vi "unmarshalling.vi"(7 "Type":variant, 8 "error in (no error)":errorcluster, 10 "B64 Encoded String":string, 11 "Serializer.Base64 in":refnum<class "Serializer.Base64.lvclass">) -> (0 "error out":errorcluster, 2 "Variant":variant, 3 "Serializer.Base64 out":refnum<class "Serializer.Base64.lvclass">)   [LabVIEW 2019, in "OpenSerializer.base64.lvlib" / "Serializer.Base64.lvclass"]
uses:
  Serializer.Base64.lvclass
  Base64_ByteLUT.vi
  <vilib>/LabVIEW Open Source Project/OpenSerializer/Serializer.FlattenedString/Serializer.FlattenedString.lvclass
  OpenSerializer.base64.lvlib
  <vilib>/LabVIEW Open Source Project/Data Manipulation/TypeDescriptor/OpenDescriptor.lvlib
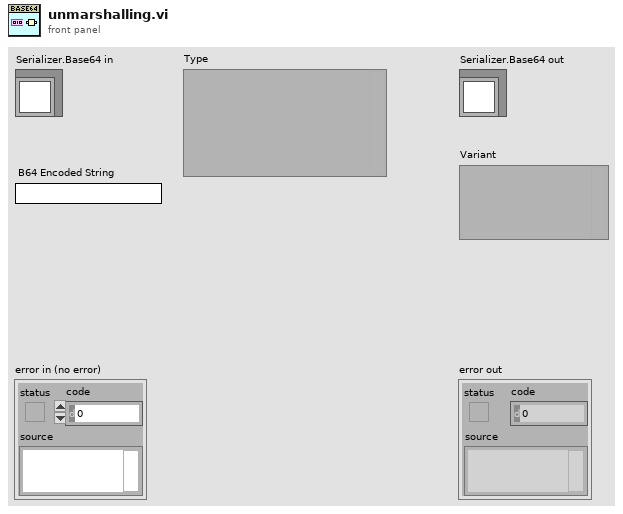
[diagram p1: front panel]
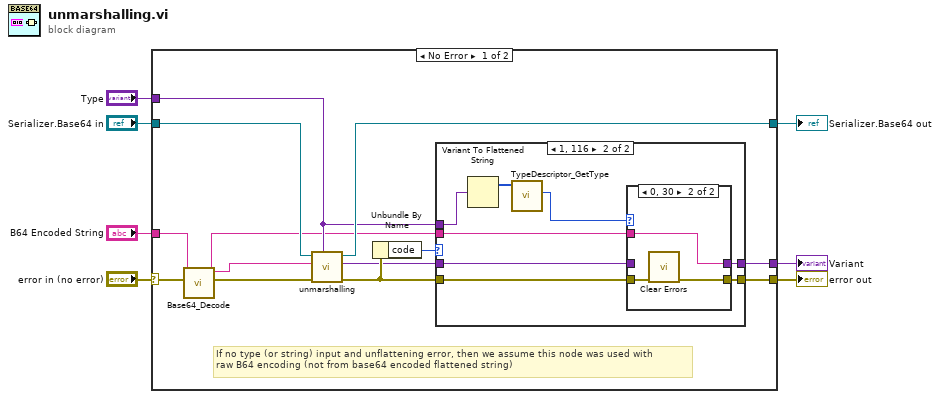
[diagram p0: block diagram]
diagram:
  n1 = case shown="No Error" "error in (no error)" {
    selector: "error in (no error)" -> [w10 w35]
    tunnel: "Serializer.Base64 in" -> [w19 w36]
    tunnel: "B64 Encoded String" -> [w9 _]
    tunnel: [w17 w36] -> w5
    tunnel: [w14 w35] -> w4
    tunnel: [w13 _] -> w3
    tunnel: "Type" -> [w11 _]
    frame No Error {
      # "If no type (or string) input and unflattening error, then we assume this node was used with\nraw B64 encoding (not from base64 encoded flattened string)"
      n2 = call "Base64_Decode.vi"("error in (no error)"=w10, "Base64 String"=w9) -> ("error out"=w18:errorcluster, "Decoded String"=w8:string)  [unwired: 8 in]
      n3 = call-parent "unmarshalling.vi"("Type"=w11, "error in (no error)"=w18, "String"=w8, "Serializer in"=w19) -> ("error out"=w15:errorcluster, "Variant"=w12:variant, "Serializer out"=w17:refnum<class "Serializer.Base64.lvclass">)  [unwired: 5 in]
      n4 = Unbundle By Name(w15) -> ("code"=w16:i32)
      n5 = case shown="1, 116" w16 {
        tunnel: w15 -> [w20 w29]
        tunnel: [w20 w28] -> w14
        tunnel: [w21 w27] -> w13
        tunnel: w12 -> [w21 w26]
        tunnel: w11 -> [_ w24]
        tunnel: w8 -> [_ w25]
        frame Default {
        }
        frame 1, 116 {
          n6 = Variant To Flattened String(Variant=w24) -> (1:w23:i16[])  [unwired: 1 out]
          n7 = call <vilib>:"TypeDescriptor_GetType.vi"("type descriptor"=w23) -> ("Type"=w22:u8)  [unwired: 9 in, 1 out]
          n8 = case shown="0, 30" w22 {
            tunnel: w29 -> [w31 w34]
            tunnel: [w31 w32] -> w28
            tunnel: [w30 w33] -> w27
            tunnel: w26 -> [w30 _]
            tunnel: w25 -> [_ w33]
            frame Default {
            }
            frame 0, 48 {
              n9 = call <vilib>:"Clear Errors.vi"("error in (no error)"=w34) -> ("error out"=w32:errorcluster)  [unwired: 5 in, 1 out]
            }
          }
        }
      }
    }
    frame Error {
    }
  }
  "error out" <- w4
  "Serializer.Base64 out" <- w5
  "Variant" <- w3
